vi "Hardware Out - NI 9759-1 (Throttle).vi"(0 "FPGA Ref":T3, 7 "ExternalAI1 (optional)":sgl, 9 "ExternalAI2 (optional)":sgl, 11 "RT Data in":T1={"Refs"={"FPGA 1"=refnum, "FPGA 2"=refnum}, "EPT"={"MaxCAD"=0.0, "EPT Sim Enabled"=FALSE, "EPTxData"={"Sync"=FALSE, "CurrentCAD"=0.0, "Speed [RPM]"=0.0, "Config"=FALSE, "Rcvg Primary"=FALSE, "Stall"=FALSE, "Overflow"=FALSE, "Ratio Error"=FALSE, "Pattern Error"=FALSE, "Aux Warning"=FALSE, "Watchdog Error"=FALSE}}, "Raw Inputs"={"NI9752s"=[], "NI9757s"=[], "NI9411s"=[], "NI9220s"=[], "VRHalls"=[]}, "Control Inputs"={"Engine Speed [RPM]"=0.0, "Engine Status"=enum."STALLED", "Load Control \nMode"=enum."Max Speed Governor", "dt(s)"=0.0, "Number of Cylinders"=0, "Engine Displacement [cc]"=0.0, "StoichAFR"=0.0, "Q.LHV Fuel [kJ/kg]"=0.0, "BattV PSU [V]"=0.0, "12V PSU [V]"=0.0, "5V PSU [V]"=0.0, "Pedal Position [%]"=0.0, "Oil Pressure [kPa]"=0.0, "Oil Temp [C]"=0.0, "Oil Level [%]"=0.0, "Engine Coolant Temp (ECT) [C]"=0.0, "Engine Coolant Pressure [kPa]"=0.0, "Rail Pressure [bar]"=0.0, "Fuel Pressure [kPa]"=0.0, "Fuel Temp [C]"=0.0, "Vacuum Pressure [kPa]"=0.0, "Throttle Position [%]"=0.0, "Cam1 Advance [CAD]"=0.0, "Cam2 Advance [CAD]"=0.0, "Cam3 Advance [CAD]"=0.0, "Cam4 Advance [CAD]"=0.0, "CA50 Control Output [CAD]"=[], "CA50 Control Output Valid"=[], "Intake Air Temp (IAT) [C]"=0.0, "Barometric Air Pressure [kPa]"=0.0, "Intake Air Rel. Humidity [%]"=0.0, "Mass Air Flow (MAF) [kg/hr]"=0.0, "Turbo Inlet Air Pressure [kPa]"=0.0, "Turbo Inlet Air Temp [C]"=0.0, "Turbo Outlet Air Pressure [kPa]"=0.0, "Turbo Outlet Air Temp [C]"=0.0, "CAC Outlet Pressure [kPa]"=0.0, "CAC Outlet Temp [C]"=0.0, "Intake Manifold Pressure (MAP) [kPa]"=0.0, "Intake Manifold Temp (MAT) [C]"=0.0, "Exhaust Manifold Pressure [kPa]"=0.0, "Exhaust Manifold Temp [C]"=0.0, "HighP EGR Cooler Outlet Pressure [kPa]"=0.0, "HighP EGR Cooler Outlet Temp [C]"=0.0, "HighP EGR Differential Pressure [kPa]"=0.0, "HighP EGR Valve Position [%]"=0.0, "Turbo Outlet Exhaust Pressure [kPa]"=0.0, "Turbo Outlet Exhaust Temp [C]"=0.0, "VGT Position 1 [%]"=0.0, "VGT Position 2 [%]"=0.0, "Turbo Speed 1 [RPM]"=0.0, "Turbo Speed 2 [RPM]"=0.0, "LowP EGR Differential Pressure [kPa]"=0.0, "LowP EGR Valve Position [%]"=0.0, "UEGO1Lambda"=0.0, "UEGO1_Hot"=FALSE, "UEGO2Lambda"=0.0, "UEGO2_Hot"=FALSE, "Knock Intensity"=[], "Knock"=[]}, "Control Outputs"={"Pedal Desired [%]"=0.0, "MEP Desired [bar]"=0.0, "Fuel Desired [mg/cyc]"=0.0, "Intake MAP Desired [kPa]"=0.0, "Cam1 Advance Setpoint [CAD]"=0.0, "Cam2 Advance Setpoint [CAD]"=0.0, "HighP EGR Position Setpoint [%Open]"=0.0, "LowP EGR Position Setpoint [%Open]"=0.0, "Rail Pressure Setpoint [bar]"=0.0, "Wastegate1 Position Setpoint [%Open]"=0.0, "Wastegate2 Position Setpoint [%Open]"=0.0, "VGT1 Position Setpoint [%Open]"=0.0, "VGT2 Position Setpoint [%Open]"=0.0, "Throttle1 Position Setpoint [%Open]"=0.0, "Throttle2 Position Setpoint [%Open]"=0.0, "TurboBPV Position Setpoint [%Open]"=0.0, "Spark Dwells [msec]"=[], "Spark Timings [DBTDC]"=[], "PFI Quantities [mg/inj]"=[], "PFI Timings [DBTDC]"=[], "DI Quantities [mg/inj]"=[], "DI Timings [DBTDC]"=[]}, "Raw Outputs"={"9751-1"={"DI1"={"Window_Start (DBTDC)"=0.0, "Window_End (DBTDC)"=0.0, "Enable_Inj1"=FALSE, "Duration_Inj1 (msec)"=0.0, "Timing_Inj1 (DBTDC)"=0.0, "Enable_Inj2"=FALSE, "Duration_Inj2 (msec)"=0.0, "Timing_Inj2 (DBTDC)"=0.0, "Enable_Inj3"=FALSE, "Duration_Inj3 (msec)"=0.0, "Timing_Inj3 (DBTDC)"=0.0, "Enable_Inj4"=FALSE, "Duration_Inj4 (msec)"=0.0, "Timing_Inj4 (DBTDC)"=0.0, "Enable_Inj5"=FALSE, "Duration_Inj5 (msec)"=0.0, "Timing_Inj5 (DBTDC)"=0.0}, "DI2"={"Window_Start (DBTDC)"=0.0, "Window_End (DBTDC)"=0.0, "Enable_Inj1"=FALSE, "Duration_Inj1 (msec)"=0.0, "Timing_Inj1 (DBTDC)"=0.0, "Enable_Inj2"=FALSE, "Duration_Inj2 (msec)"=0.0, "Timing_Inj2 (DBTDC)"=0.0, "Enable_Inj3"=FALSE, "Duration_Inj3 (msec)"=0.0, "Timing_Inj3 (DBTDC)"=0.0, "Enable_Inj4"=FALSE, "Duration_Inj4 (msec)"=0.0, "Timing_Inj4 (DBTDC)"=0.0, "Enable_Inj5"=FALSE, "Duration_Inj5 (msec)"=0.0, "Timing_Inj5 (DBTDC)"=0.0}, "DI3"={"Window_Start (DBTDC)"=0.0, "Window_End (DBTDC)"=0.0, "Enable_Inj1"=FALSE, "Duration_Inj1 (msec)"=0.0, "Timing_Inj1 (DBTDC)"=0.0, "Enable_Inj2"=FALSE, "Duration_Inj2 (msec)"=0.0, "Timing_Inj2 (DBTDC)"=0.0, "Enable_Inj3"=FALSE, "Duration_Inj3 (msec)"=0.0, "Timing_Inj3 (DBTDC)"=0.0, "Enable_Inj4"=FALSE, "Duration_Inj4 (msec)"=0.0, "Timing_Inj4 (DBTDC)"=0.0, "Enable_Inj5"=FALSE, "Duration_Inj5 (msec)"=0.0, "Timing_Inj5 (DBTDC)"=0.0}}, "9751-2"={"DI1"={"Window_Start (DBTDC)"=0.0, "Window_End (DBTDC)"=0.0, "Enable_Inj1"=FALSE, "Duration_Inj1 (msec)"=0.0, "Timing_Inj1 (DBTDC)"=0.0, "Enable_Inj2"=FALSE, "Duration_Inj2 (msec)"=0.0, "Timing_Inj2 (DBTDC)"=0.0, "Enable_Inj3"=FALSE, "Duration_Inj3 (msec)"=0.0, "Timing_Inj3 (DBTDC)"=0.0, "Enable_Inj4"=FALSE, "Duration_Inj4 (msec)"=0.0, "Timing_Inj4 (DBTDC)"=0.0, "Enable_Inj5"=FALSE, "Duration_Inj5 (msec)"=0.0, "Timing_Inj5 (DBTDC)"=0.0}, "DI2"={"Window_Start (DBTDC)"=0.0, "Window_End (DBTDC)"=0.0, "Enable_Inj1"=FALSE, "Duration_Inj1 (msec)"=0.0, "Timing_Inj1 (DBTDC)"=0.0, "Enable_Inj2"=FALSE, "Duration_Inj2 (msec)"=0.0, "Timing_Inj2 (DBTDC)"=0.0, "Enable_Inj3"=FALSE, "Duration_Inj3 (msec)"=0.0, "Timing_Inj3 (DBTDC)"=0.0, "Enable_Inj4"=FALSE, "Duration_Inj4 (msec)"=0.0, "Timing_Inj4 (DBTDC)"=0.0, "Enable_Inj5"=FALSE, "Duration_Inj5 (msec)"=0.0, "Timing_Inj5 (DBTDC)"=0.0}, "DI3"={"Window_Start (DBTDC)"=0.0, "Window_End (DBTDC)"=0.0, "Enable_Inj1"=FALSE, "Duration_Inj1 (msec)"=0.0, "Timing_Inj1 (DBTDC)"=0.0, "Enable_Inj2"=FALSE, "Duration_Inj2 (msec)"=0.0, "Timing_Inj2 (DBTDC)"=0.0, "Enable_Inj3"=FALSE, "Duration_Inj3 (msec)"=0.0, "Timing_Inj3 (DBTDC)"=0.0, "Enable_Inj4"=FALSE, "Duration_Inj4 (msec)"=0.0, "Timing_Inj4 (DBTDC)"=0.0, "Enable_Inj5"=FALSE, "Duration_Inj5 (msec)"=0.0, "Timing_Inj5 (DBTDC)"=0.0}}, "9751-3"={"DI1"={"Window_Start (DBTDC)"=0.0, "Window_End (DBTDC)"=0.0, "Enable_Inj1"=FALSE, "Duration_Inj1 (msec)"=0.0, "Timing_Inj1 (DBTDC)"=0.0, "Enable_Inj2"=FALSE, "Duration_Inj2 (msec)"=0.0, "Timing_Inj2 (DBTDC)"=0.0, "Enable_Inj3"=FALSE, "Duration_Inj3 (msec)"=0.0, "Timing_Inj3 (DBTDC)"=0.0, "Enable_Inj4"=FALSE, "Duration_Inj4 (msec)"=0.0, "Timing_Inj4 (DBTDC)"=0.0, "Enable_Inj5"=FALSE, "Duration_Inj5 (msec)"=0.0, "Timing_Inj5 (DBTDC)"=0.0}, "DI2"={"Window_Start (DBTDC)"=0.0, "Window_End (DBTDC)"=0.0, "Enable_Inj1"=FALSE, "Duration_Inj1 (msec)"=0.0, "Timing_Inj1 (DBTDC)"=0.0, "Enable_Inj2"=FALSE, "Duration_Inj2 (msec)"=0.0, "Timing_Inj2 (DBTDC)"=0.0, "Enable_Inj3"=FALSE, "Duration_Inj3 (msec)"=0.0, "Timing_Inj3 (DBTDC)"=0.0, "Enable_Inj4"=FALSE, "Duration_Inj4 (msec)"=0.0, "Timing_Inj4 (DBTDC)"=0.0, "Enable_Inj5"=FALSE, "Duration_Inj5 (msec)"=0.0, "Timing_Inj5 (DBTDC)"=0.0}, "DI3"={"Window_Start (DBTDC)"=0.0, "Window_End (DBTDC)"=0.0, "Enable_Inj1"=FALSE, "Duration_Inj1 (msec)"=0.0, "Timing_Inj1 (DBTDC)"=0.0, "Enable_Inj2"=FALSE, "Duration_Inj2 (msec)"=0.0, "Timing_Inj2 (DBTDC)"=0.0, "Enable_Inj3"=FALSE, "Duration_Inj3 (msec)"=0.0, "Timing_Inj3 (DBTDC)"=0.0, "Enable_Inj4"=FALSE, "Duration_Inj4 (msec)"=0.0, "Timing_Inj4 (DBTDC)"=0.0, "Enable_Inj5"=FALSE, "Duration_Inj5 (msec)"=0.0, "Timing_Inj5 (DBTDC)"=0.0}}, "9751-4"={"DI1"={"Window_Start (DBTDC)"=0.0, "Window_End (DBTDC)"=0.0, "Enable_Inj1"=FALSE, "Duration_Inj1 (msec)"=0.0, "Timing_Inj1 (DBTDC)"=0.0, "Enable_Inj2"=FALSE, "Duration_Inj2 (msec)"=0.0, "Timing_Inj2 (DBTDC)"=0.0, "Enable_Inj3"=FALSE, "Duration_Inj3 (msec)"=0.0, "Timing_Inj3 (DBTDC)"=0.0, "Enable_Inj4"=FALSE, "Duration_Inj4 (msec)"=0.0, "Timing_Inj4 (DBTDC)"=0.0, "Enable_Inj5"=FALSE, "Duration_Inj5 (msec)"=0.0, "Timing_Inj5 (DBTDC)"=0.0}, "DI2"={"Window_Start (DBTDC)"=0.0, "Window_End (DBTDC)"=0.0, "Enable_Inj1"=FALSE, "Duration_Inj1 (msec)"=0.0, "Timing_Inj1 (DBTDC)"=0.0, "Enable_Inj2"=FALSE, "Duration_Inj2 (msec)"=0.0, "Timing_Inj2 (DBTDC)"=0.0, "Enable_Inj3"=FALSE, "Duration_Inj3 (msec)"=0.0, "Timing_Inj3 (DBTDC)"=0.0, "Enable_Inj4"=FALSE, "Duration_Inj4 (msec)"=0.0, "Timing_Inj4 (DBTDC)"=0.0, "Enable_Inj5"=FALSE, "Duration_Inj5 (msec)"=0.0, "Timing_Inj5 (DBTDC)"=0.0}, "DI3"={"Window_Start (DBTDC)"=0.0, "Window_End (DBTDC)"=0.0, "Enable_Inj1"=FALSE, "Duration_Inj1 (msec)"=0.0, "Timing_Inj1 (DBTDC)"=0.0, "Enable_Inj2"=FALSE, "Duration_Inj2 (msec)"=0.0, "Timing_Inj2 (DBTDC)"=0.0, "Enable_Inj3"=FALSE, "Duration_Inj3 (msec)"=0.0, "Timing_Inj3 (DBTDC)"=0.0, "Enable_Inj4"=FALSE, "Duration_Inj4 (msec)"=0.0, "Timing_Inj4 (DBTDC)"=0.0, "Enable_Inj5"=FALSE, "Duration_Inj5 (msec)"=0.0, "Timing_Inj5 (DBTDC)"=0.0}}, "9754-1"={"ESTTL 1"={"Timing (DBTDC)"=0.0, "Dwell (ms)"=0.0}, "ESTTL 2"={"Timing (DBTDC)"=0.0, "Dwell (ms)"=0.0}, "ESTTL 3"={"Timing (DBTDC)"=0.0, "Dwell (ms)"=0.0}, "ESTTL 4"={"Timing (DBTDC)"=0.0, "Dwell (ms)"=0.0}, "ESTTL 5"={"Timing (DBTDC)"=0.0, "Dwell (ms)"=0.0}, "ESTTL 6"={"Timing (DBTDC)"=0.0, "Dwell (ms)"=0.0}, "ESTTL 7"={"Timing (DBTDC)"=0.0, "Dwell (ms)"=0.0}, "ESTTL 8"={"Timing (DBTDC)"=0.0, "Dwell (ms)"=0.0}}, "9754-2"={"ESTTL 1"={"Timing (DBTDC)"=0.0, "Dwell (ms)"=0.0}, "ESTTL 2"={"Timing (DBTDC)"=0.0, "Dwell (ms)"=0.0}, "ESTTL 3"={"Timing (DBTDC)"=0.0, "Dwell (ms)"=0.0}, "ESTTL 4"={"Timing (DBTDC)"=0.0, "Dwell (ms)"=0.0}, "ESTTL 5"={"Timing (DBTDC)"=0.0, "Dwell (ms)"=0.0}, "ESTTL 6"={"Timing (DBTDC)"=0.0, "Dwell (ms)"=0.0}, "ESTTL 7"={"Timing (DBTDC)"=0.0, "Dwell (ms)"=0.0}, "ESTTL 8"={"Timing (DBTDC)"=0.0, "Dwell (ms)"=0.0}}, "9758-1"={"LS 1"={"Enable"=FALSE, "Freq [Hz]"=0.0, "DutyCyc [%]"=0.0}, "LS 2"={"Enable"=FALSE, "Freq [Hz]"=0.0, "DutyCyc [%]"=0.0}, "LS 3"={"Enable"=FALSE, "Freq [Hz]"=0.0, "DutyCyc [%]"=0.0}, "LS 4"={"Enable"=FALSE, "Freq [Hz]"=0.0, "DutyCyc [%]"=0.0}, "PFI 1"={"Position Mode"=FALSE, "Timing (DBTDC)"=0.0, "Pulse Width (ms)"=0.0}, "PFI 2"={"Position Mode"=FALSE, "Timing (DBTDC)"=0.0, "Pulse Width (ms)"=0.0}, "PFI 3"={"Position Mode"=FALSE, "Timing (DBTDC)"=0.0, "Pulse Width (ms)"=0.0}, "PFI 4"={"Position Mode"=FALSE, "Timing (DBTDC)"=0.0, "Pulse Width (ms)"=0.0}}, "9758-2"={"LS 1"={"Enable"=FALSE, "Freq [Hz]"=0.0, "DutyCyc [%]"=0.0}, "LS 2"={"Enable"=FALSE, "Freq [Hz]"=0.0, "DutyCyc [%]"=0.0}, "LS 3"={"Enable"=FALSE, "Freq [Hz]"=0.0, "DutyCyc [%]"=0.0}, "LS 4"={"Enable"=FALSE, "Freq [Hz]"=0.0, "DutyCyc [%]"=0.0}, "PFI 1"={"Position Mode"=FALSE, "Timing (DBTDC)"=0.0, "Pulse Width (ms)"=0.0}, "PFI 2"={"Position Mode"=FALSE, "Timing (DBTDC)"=0.0, "Pulse Width (ms)"=0.0}, "PFI 3"={"Position Mode"=FALSE, "Timing (DBTDC)"=0.0, "Pulse Width (ms)"=0.0}, "PFI 4"={"Position Mode"=FALSE, "Timing (DBTDC)"=0.0, "Pulse Width (ms)"=0.0}}, "9759-1"={"THR1-1 DC [%]"=0.0, "THR1-1 Setpoint [% Open]"=0.0, "THR1-2 DC [%]"=0.0, "THR1-2 Setpoint [% Open]"=0.0}}} {"Control Inputs"."Knock Intensity" format="%.2f"; "Control Inputs"."CA50 Control Output [CAD]" format="%.2f"; "Control Inputs"."Exhaust Manifold Temp [C]" format="%#_6f"; "Control Inputs"."UEGO2Lambda" format="%.2f"; "Control Inputs"."Intake Manifold Temp (MAT) [C]" format="%#_6f"; "Control Inputs"."UEGO1Lambda" format="%.2f"}) -> ()   [LabVIEW 2015, in "ECS-RT.lvlib"]
uses:
  ECS-RT.lvlib
  Typedefs/FPGA Refs/Generic FPGA Ref.ctl
  Typedefs/RT Data.ctl
  Typedefs/FPGA Refs/FPGA Refs.ctl
  Typedefs/EPT/EPT Cluster.ctl
  <vilib>/Powertrain Controls/Device Drivers/Engine Position Tracking/EPTx/RevA/RT/Controls/EPTxData.ctl
  Typedefs/Raw Inputs/Raw Inputs.ctl
  Typedefs/Raw Inputs/NI9752.ctl
  Typedefs/Raw Inputs/PPWData.ctl
  Typedefs/Raw Inputs/NI9757.ctl
  Typedefs/Raw Inputs/NI9411.ctl
  Typedefs/Raw Inputs/NI9220.ctl
  Typedefs/Raw Inputs/VRHall.ctl
  Typedefs/Control Inputs/Control Inputs.ctl
  Typedefs/EPT/Engine Status.ctl
  Typedefs/MISC/Load Control Mode.ctl
  Typedefs/Control Outputs/Control Outputs.ctl
  Typedefs/Control Outputs/Injection Quantity.ctl
  Typedefs/Control Outputs/Injection Timing.ctl
  Typedefs/Raw Outputs/Raw Outputs.ctl
  Typedefs/Raw Outputs/NI9751.ctl
  Typedefs/Raw Outputs/DI.ctl
  Typedefs/Raw Outputs/NI9754.ctl
  Typedefs/Raw Outputs/ESTTL.ctl
  Typedefs/Raw Outputs/NI9758.ctl
  Typedefs/Raw Outputs/LS.ctl
  Typedefs/Raw Outputs/PFI.ctl
  Typedefs/Raw Outputs/NI9759.ctl
  <vilib>/Powertrain Controls/Device Drivers/Throttle/RevB2/Real-Time/Support/Mode Request.ctl
  <vilib>/Utility/error.llb/Error Cluster From Error Code.vi
  <vilib>/rvi/errors/niLvFpgaAdjustHostInterfaceError.vi
  <vilib>/rvi/interface/nirviReadWriteControl/nirviReadWriteControl.xnode
  <vilib>/rvi/interface/Simulation/niFpgaSimulationCallBeginRW.vi
  NiFpgaLv.dll
  ECS-Shared.lvlib
  <vilib>/Powertrain Controls/Device Drivers/Engine Position Tracking/EPTx/RevA/RT/EPTx - RevA - RT.lvlib
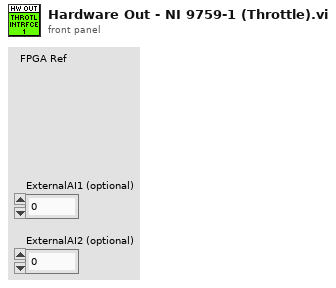
[diagram p1: front panel]
types:
  T1 = typedef "ECS-Shared.lvlib/RT Data.ctl" = cluster{"Refs":T2, "EPT":T4, "Raw Inputs":T6, "Control Inputs":T13, "Control Outputs":T16, "Raw Outputs":T19}
  T2 = typedef "ECS-Shared.lvlib/FPGA Refs.ctl" = cluster{"FPGA 1":T3, "FPGA 2":T3}
  T3 = typedef "ECS-Shared.lvlib/Generic FPGA Ref.ctl" = refnum<k20>
  T4 = typedef "ECS-Shared.lvlib/EPT Cluster.ctl" = cluster{"MaxCAD":sgl, "EPT Sim Enabled":bool, "EPTxData":T5}
  T5 = typedef "EPTx - RevA - RT.lvlib/EPTxData.ctl" = cluster{"Sync":bool, "CurrentCAD":sgl, "Speed [RPM]":sgl, "Config":bool, "Rcvg Primary":bool, "Stall":bool, "Overflow":bool, "Ratio Error":bool, "Pattern Error":bool, "Aux Warning":bool, "Watchdog Error":bool}
  T6 = typedef "ECS-Shared.lvlib/Raw Inputs.ctl" = cluster{"NI9752s":T7[], "NI9757s":T9[], "NI9411s":T10[], "NI9220s":T11[], "VRHalls":T12[]}
  T7 = typedef "ECS-Shared.lvlib/NI9752.ctl" = cluster{"Voltage [V]":sgl[], "Resistance [Ohm]":sgl[], "PPWData VR1":T8, "PPWData VR2":T8, "PPWData Hall1":T8, "PPWData Hall2":T8}
  T8 = typedef "ECS-Shared.lvlib/PPWData.ctl" = cluster{"Period":u32, "PulseWidth":u32, "Stopped":bool}
  T9 = typedef "ECS-Shared.lvlib/NI9757.ctl" = cluster{"UEGO1":cluster{"Lambda":sgl, "Phi":sgl, "AF_Ratio":sgl, "Ip":sgl, "Temp":sgl, "Hot":bool}, "UEGO2":cluster{"Lambda":sgl, "Phi":sgl, "AF_Ratio":sgl, "Ip":sgl, "Temp":sgl, "Hot":bool}, "EGO1":cluster{"Status":enum16{"COLD SENSOR", "FOULED SENSOR", "RICH", "LEAN"}, "SensorV":sgl}, "EGO2":cluster{"Status":enum16{"COLD SENSOR", "FOULED SENSOR", "RICH", "LEAN"}, "SensorV":sgl}, "EGO3":cluster{"Status":enum16{"COLD SENSOR", "FOULED SENSOR", "RICH", "LEAN"}, "SensorV":sgl}, "EGO4":cluster{"Status":enum16{"COLD SENSOR", "FOULED SENSOR", "RICH", "LEAN"}, "SensorV":sgl}}
  T10 = typedef "ECS-Shared.lvlib/NI9411.ctl" = cluster{"PPWData 0":T8, "PPWData 1":T8, "PPWData 2":T8, "PPWData 3":T8, "PPWData 4":T8, "PPWData 5":T8}
  T11 = typedef "ECS-Shared.lvlib/NI9220.ctl" = cluster{"AI 0":sgl, "AI 1":sgl, "AI 2":sgl, "AI 3":sgl, "AI 4":sgl, "AI 5":sgl, "AI 6":sgl, "AI 7":sgl, "AI 8":sgl, "AI 9":sgl, "AI 10":sgl, "AI 11":sgl, "AI 12":sgl, "AI 13":sgl, "AI 14":sgl, "AI 15":sgl}
  T12 = typedef "ECS-Shared.lvlib/VRHall.ctl" = cluster{"PPWData 0":T8, "PPWData 1":T8, "PPWData 2":T8, "PPWData 3":T8, "PPWData 4":T8, "PPWData 5":T8}
  T13 = typedef "ECS-Shared.lvlib/Control Inputs.ctl" = cluster{"Engine Speed [RPM]":sgl, "Engine Status":T14, "Load Control \nMode":T15, "dt(s)":sgl, "Number of Cylinders":u8, "Engine Displacement [cc]":sgl, "StoichAFR":sgl, "Q.LHV Fuel [kJ/kg]":sgl, "BattV PSU [V]":sgl, "12V PSU [V]":sgl, "5V PSU [V]":sgl, "Pedal Position [%]":sgl, "Oil Pressure [kPa]":sgl, "Oil Temp [C]":sgl, "Oil Level [%]":sgl, "Engine Coolant Temp (ECT) [C]":sgl, "Engine Coolant Pressure [kPa]":sgl, "Rail Pressure [bar]":sgl, "Fuel Pressure [kPa]":sgl, "Fuel Temp [C]":sgl, "Vacuum Pressure [kPa]":sgl, "Throttle Position [%]":sgl, "Cam1 Advance [CAD]":sgl, "Cam2 Advance [CAD]":sgl, "Cam3 Advance [CAD]":sgl, "Cam4 Advance [CAD]":sgl, "CA50 Control Output [CAD]":sgl[], "CA50 Control Output Valid":bool[], "Intake Air Temp (IAT) [C]":sgl, "Barometric Air Pressure [kPa]":sgl, "Intake Air Rel. Humidity [%]":sgl, "Mass Air Flow (MAF) [kg/hr]":sgl, "Turbo Inlet Air Pressure [kPa]":sgl, "Turbo Inlet Air Temp [C]":sgl, "Turbo Outlet Air Pressure [kPa]":sgl, "Turbo Outlet Air Temp [C]":sgl, "CAC Outlet Pressure [kPa]":sgl, "CAC Outlet Temp [C]":sgl, "Intake Manifold Pressure (MAP) [kPa]":sgl, "Intake Manifold Temp (MAT) [C]":sgl, "Exhaust Manifold Pressure [kPa]":sgl, "Exhaust Manifold Temp [C]":sgl, "HighP EGR Cooler Outlet Pressure [kPa]":sgl, "HighP EGR Cooler Outlet Temp [C]":sgl, "HighP EGR Differential Pressure [kPa]":sgl, "HighP EGR Valve Position [%]":sgl, "Turbo Outlet Exhaust Pressure [kPa]":sgl, "Turbo Outlet Exhaust Temp [C]":sgl, "VGT Position 1 [%]":sgl, "VGT Position 2 [%]":sgl, "Turbo Speed 1 [RPM]":sgl, "Turbo Speed 2 [RPM]":sgl, "LowP EGR Differential Pressure [kPa]":sgl, "LowP EGR Valve Position [%]":sgl, "UEGO1Lambda":sgl, "UEGO1_Hot":bool, "UEGO2Lambda":sgl, "UEGO2_Hot":bool, "Knock Intensity":sgl[], "Knock":bool[]}
  T14 = typedef "ECS-Shared.lvlib/Engine Status.ctl" = enum16{"OFF", "STALLED", "CRANKING", "RUNNING", "ACCEL", "DECEL", "SAFE"}
  T15 = typedef "ECS-Shared.lvlib/Load Control Mode.ctl" = enum16{"No Governor", "Min Speed Governor", "Max Speed Governor"}
  T16 = typedef "ECS-Shared.lvlib/Control Outputs.ctl" = cluster{"Pedal Desired [%]":sgl, "MEP Desired [bar]":sgl, "Fuel Desired [mg/cyc]":sgl, "Intake MAP Desired [kPa]":sgl, "Cam1 Advance Setpoint [CAD]":sgl, "Cam2 Advance Setpoint [CAD]":sgl, "HighP EGR Position Setpoint [%Open]":sgl, "LowP EGR Position Setpoint [%Open]":sgl, "Rail Pressure Setpoint [bar]":sgl, "Wastegate1 Position Setpoint [%Open]":sgl, "Wastegate2 Position Setpoint [%Open]":sgl, "VGT1 Position Setpoint [%Open]":sgl, "VGT2 Position Setpoint [%Open]":sgl, "Throttle1 Position Setpoint [%Open]":sgl, "Throttle2 Position Setpoint [%Open]":sgl, "TurboBPV Position Setpoint [%Open]":sgl, "Spark Dwells [msec]":sgl[], "Spark Timings [DBTDC]":sgl[], "PFI Quantities [mg/inj]":sgl[], "PFI Timings [DBTDC]":sgl[], "DI Quantities [mg/inj]":T17[], "DI Timings [DBTDC]":T18[]}
  T17 = typedef "ECS-Shared.lvlib/Injection Quantity.ctl" = cluster{"Pilot1Quantity [mg/inj]":sgl, "Pilot2Quantity [mg/inj]":sgl, "MainQuantity [mg/inj]":sgl, "Post1Quantity [mg/inj]":sgl, "Post2Quantity [mg/inj]":sgl}
  T18 = typedef "ECS-Shared.lvlib/Injection Timing.ctl" = cluster{"Pilot1SOI [DBTDC]":sgl, "Pilot2SOI [DBTDC]":sgl, "MainSOI [DBTDC]":sgl, "Post1SOI [DBTDC]":sgl, "Post2SOI [DBTDC]":sgl}
  T19 = typedef "ECS-Shared.lvlib/Raw Outputs.ctl" = cluster{"9751-1":T20, "9751-2":T20, "9751-3":T20, "9751-4":T20, "9754-1":T22, "9754-2":T22, "9758-1":T24, "9758-2":T24, "9759-1":T27}
  T20 = typedef "ECS-Shared.lvlib/NI9751.ctl" = cluster{"DI1":T21, "DI2":T21, "DI3":T21}
  T21 = typedef "ECS-Shared.lvlib/DI.ctl" = cluster{"Window_Start (DBTDC)":sgl, "Window_End (DBTDC)":sgl, "Enable_Inj1":bool, "Duration_Inj1 (msec)":sgl, "Timing_Inj1 (DBTDC)":sgl, "Enable_Inj2":bool, "Duration_Inj2 (msec)":sgl, "Timing_Inj2 (DBTDC)":sgl, "Enable_Inj3":bool, "Duration_Inj3 (msec)":sgl, "Timing_Inj3 (DBTDC)":sgl, "Enable_Inj4":bool, "Duration_Inj4 (msec)":sgl, "Timing_Inj4 (DBTDC)":sgl, "Enable_Inj5":bool, "Duration_Inj5 (msec)":sgl, "Timing_Inj5 (DBTDC)":sgl}
  T22 = typedef "ECS-Shared.lvlib/NI9754.ctl" = cluster{"ESTTL 1":T23, "ESTTL 2":T23, "ESTTL 3":T23, "ESTTL 4":T23, "ESTTL 5":T23, "ESTTL 6":T23, "ESTTL 7":T23, "ESTTL 8":T23}
  T23 = typedef "ECS-Shared.lvlib/ESTTL.ctl" = cluster{"Timing (DBTDC)":sgl, "Dwell (ms)":sgl}
  T24 = typedef "ECS-Shared.lvlib/NI9758.ctl" = cluster{"LS 1":T25, "LS 2":T25, "LS 3":T25, "LS 4":T25, "PFI 1":T26, "PFI 2":T26, "PFI 3":T26, "PFI 4":T26}
  T25 = typedef "ECS-Shared.lvlib/LS.ctl" = cluster{"Enable":bool, "Freq [Hz]":sgl, "DutyCyc [%]":sgl}
  T26 = typedef "ECS-Shared.lvlib/PFI.ctl" = cluster{"Position Mode":bool, "Timing (DBTDC)":sgl, "Pulse Width (ms)":sgl}
  T27 = typedef "ECS-Shared.lvlib/NI9759.ctl" = cluster{"THR1-1 DC [%]":sgl, "THR1-1 Setpoint [% Open]":sgl, "THR1-2 DC [%]":sgl, "THR1-2 Setpoint [% Open]":sgl}
  T28 = cluster{"TLead (sec)":sgl, "TLag (sec)":sgl, "KRpos (V/ )":sgl, "TIpos (sec)":sgl, "TDpos (sec)":sgl, "KRneg (V/ )":sgl, "TIneg (sec)":sgl, "TDneg (sec)":sgl, "LH Position Band":sgl, "U LH (V)":sgl, "U LH Lag (sec)":sgl, "US (V)":sgl, "US Lag (sec)":sgl, "LH Position":sgl, "Motor Resistance (Ohms)":sgl, "Position Fault Thresh":sgl}
  T29 = typedef "Mode Request.ctl" = enum16{"IDLE", "POSITION CALIBRATION", "CONTROL CALIBRATION", "CONTROL"}
  T30 = cluster{"Analog1 Range (V)":sgl[], "Analog2 Range (V)":sgl[], "Position Range":sgl[]}
  T31 = cluster{"Psn Cal Init Delay (sec)":sgl, "Psn Cal Return From Postive Delay (sec)":sgl, "Psn Cal Return From Negative Delay (sec)":sgl, "u Psn Cal Postive Init (V)":sgl, "u Psn Cal Negative Init (V)":sgl, "u Psn Cal Inc (V)":sgl, "u Psn Cal Dec (V)":sgl, "u Psn Cal Inc Thresh (V)":sgl, "u Psn Cal Dec Thresh (V)":sgl, "Psn Cal Offset (V)":sgl, "Psn Cal Diff Thresh (V)":sgl}
  T32 = cluster{"ModuleEnable":bool, "WatchdogIn":bool, "ThrottlePeriod":u16, "Throttle2Period":u16, "ThrottlePulseWidth":i16, "Throttle2PulseWidth":i16}
  T33 = cluster{"ModulePresent":bool, "H1Sense":i16, "H2Sense":i16, "Analog1":i16, "Analog2":i16, "Battery":i16, "Temperature":i16, "Fault1":bool, "Fault2":bool}
  T34 = cluster{"ModulePresent":bool, "H1Sense (A)":sgl, "H2Sense (A)":sgl, "Analog1 (V)":sgl, "Analog2 (V)":sgl, "Battery (V)":sgl, "Temperature (C)":sgl, "H1Fault":bool, "H2Fault":bool}
  T35 = cluster{"Primary Analog Range (V)":sgl[], "Secondary Analog Range (V)":sgl[], "Position Range":sgl[], "Position Calibrated":bool, "u Pos Cal Positive (V)":sgl, "u Pos Cal Negative (V)":sgl, "u Limit Positive":bool, "u Limit Negative":bool, "Pos Cal Diff Fault":bool}
  T36 = typedef "Mode Status.ctl" = enum16{"IDLE", "POSITION CALIBRATION", "CONTROL CALIBRATION", "CONTROL"}
  T37 = cluster{"Primary Position":sgl, "Secondary Position":sgl, "AboveLH?":bool, "Position Fault":bool, "u Limit?":bool, "uLHc (V)":sgl, "uFc (V)":sgl, "uPID (V)":sgl, "u (V)":sgl}
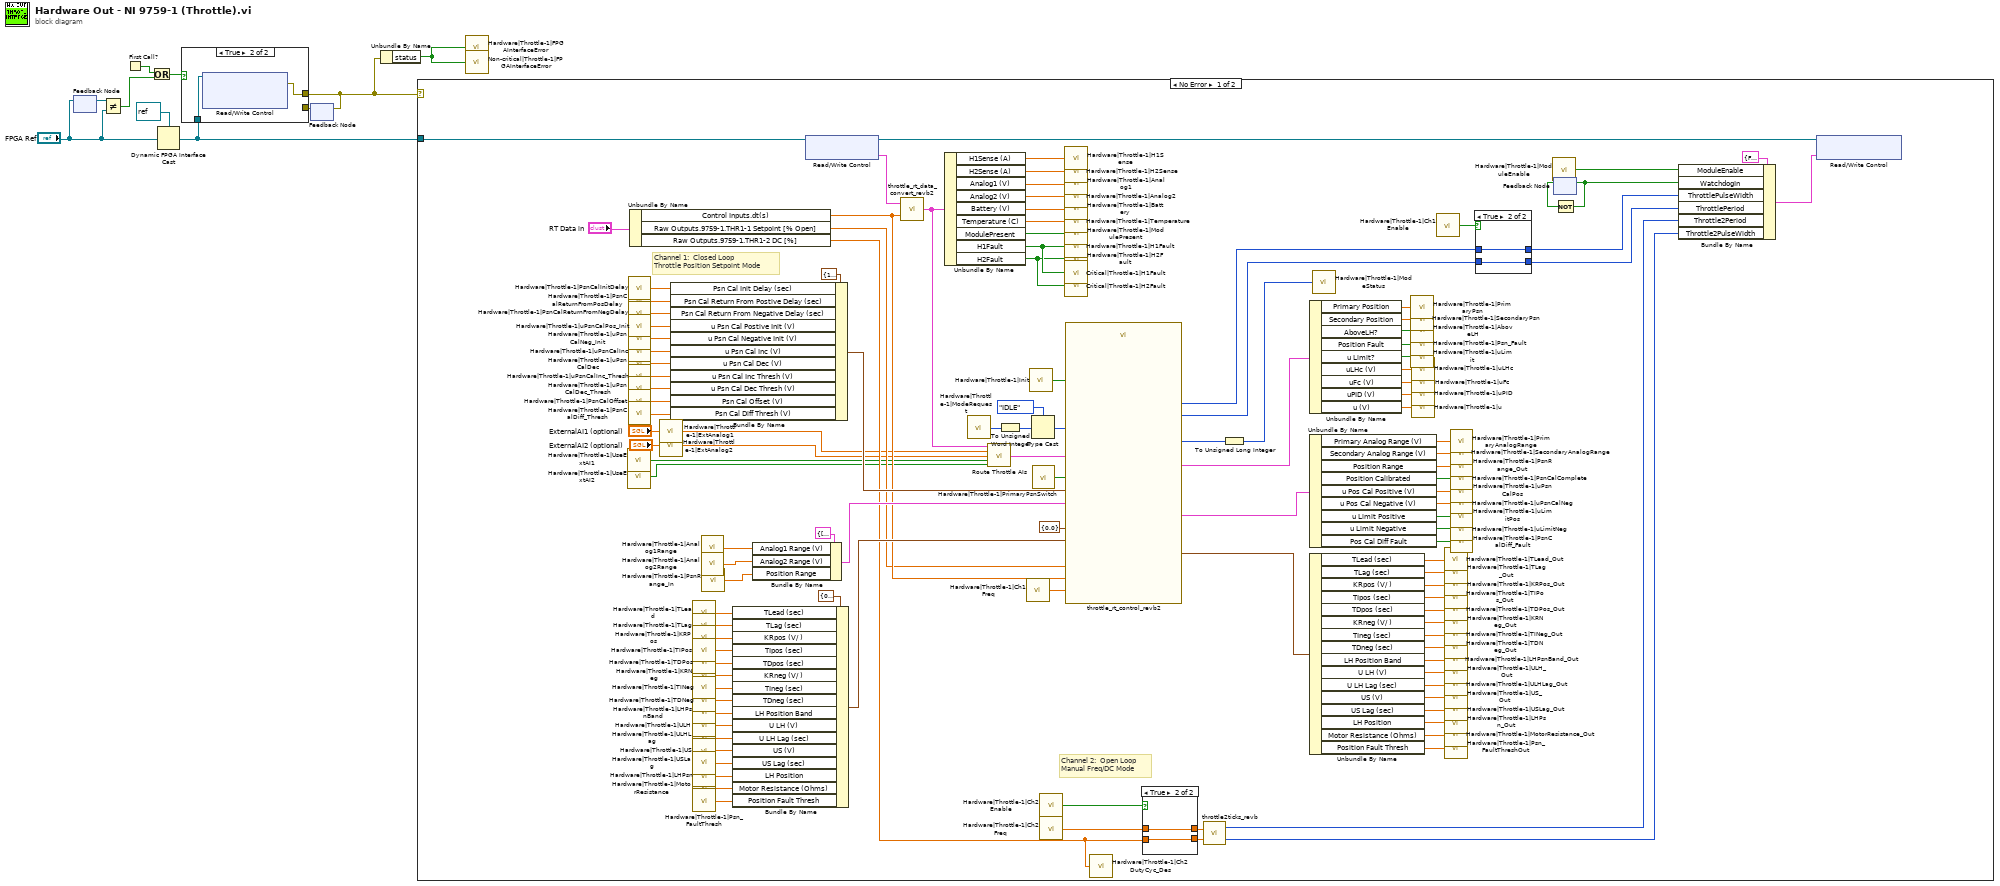
[diagram p0: block diagram]
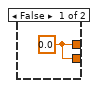
[diagram p3: hidden frame]
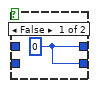
[diagram p4: hidden frame]
diagram:
  n1 = feedback #1() -> (w7:T3)  [unwired: 1 in]
  n2 = feedback-in #1("FPGA Ref") -> ()
  n3 = Not Equal?(x=w7, y="FPGA Ref") -> (x != y?=w6:bool)
  n4 = First Call?() -> (First Call?: T/F=w8:bool)
  n5 = Or(x=w8, y=w6) -> (x .or. y?=w9:bool)
  n6 = Dynamic FPGA Interface Cast(Session In=refnum<k20> refnum ("NI 9759 (Throttle)"), Type="FPGA Ref") -> (Session Out=w5:refnum<k20>)
  n7 = feedback #2() -> (w10:errorcluster)  [unwired: 1 in]
  n8 = case shown="True" w9 {
    tunnel: [w11 w13] -> w2
    tunnel: w10 -> [w11 _]
    tunnel: w5 -> [_ w12]
    frame False {
    }
    frame True {
      n9 = xnode "Read/Write Control"("FPGA VI Reference In"=w12) -> ("error out"=w13:errorcluster)  [unwired: 2 in, 2 out]
    }
  }
  n10 = feedback-in #2(w2) -> ()
  n11 = Unbundle By Name(w2) -> ("status"=w1:bool)
  n12 = case shown="No Error" w2 {
    tunnel: w5 -> [w27 _]
    frame No Error {
      # "Channel 2:  Open Loop\nManual Freq/DC Mode"
      # "Channel 1:  Closed Loop\nThrottle Position Setpoint Mode"
      n13 = call "Hardware|Throttle-1|UseExtAI1"() -> ("Value"=w17:bool)
      n14 = call "Hardware|Throttle-1|UseExtAI2"() -> ("Value"=w16:bool)
      n15 = call "Hardware|Throttle-1|PsnCalInitDelay"() -> ("Value"=w106:sgl)
      n16 = call "Hardware|Throttle-1|PsnCalReturnFromPosDelay"() -> ("Value"=w104:sgl)
      n17 = call "Hardware|Throttle-1|PsnCalReturnFromNegDelay"() -> ("Value"=w103:sgl)
      n18 = call "Hardware|Throttle-1|uPsnCalPos_Init"() -> ("Value"=w102:sgl)
      n19 = call "Hardware|Throttle-1|uPsnCalNeg_Init"() -> ("Value"=w101:sgl)
      n20 = call "Hardware|Throttle-1|uPsnCalInc"() -> ("Value"=w100:sgl)
      n21 = call "Hardware|Throttle-1|uPsnCalDec"() -> ("Value"=w99:sgl)
      n22 = call "Hardware|Throttle-1|uPsnCalInc_Thresh"() -> ("Value"=w98:sgl)
      n23 = call "Hardware|Throttle-1|uPsnCalDec_Thresh"() -> ("Value"=w97:sgl)
      n24 = call "Hardware|Throttle-1|PsnCalOffset"() -> ("Value"=w96:sgl)
      n25 = call "Hardware|Throttle-1|PsnCalDiff_Thresh"() -> ("Value"=w105:sgl)
      n26 = Unbundle By Name("RT Data in") -> ("Control Inputs.dt(s)"=w23:sgl, "Raw Outputs.9759-1.THR1-1 Setpoint [% Open]"=w22:sgl, "Raw Outputs.9759-1.THR1-2 DC [%]"=w21:sgl)
      n27 = call "Hardware|Throttle-1|ExtAnalog1"("Value"="ExternalAI1 (optional)") -> ()
      n28 = call "Hardware|Throttle-1|ExtAnalog2"("Value"="ExternalAI2 (optional)") -> ()
      n29 = Bundle By Name(cluster=T31 {"Psn Cal Init Delay (sec)"=1.0, "Psn Cal Return From Postive Delay (sec)"=1.0, "Psn Cal Return From Negative Delay (sec)"=1.0, "u Psn Cal Postive Init (V)"=3.4, "u Psn Cal Negative Init (V)"=-3.0, "u Psn Cal Inc (V)"=0.2, "u Psn Cal Dec (V)"=-0.2, "u Psn Cal Inc Thresh (V)"=1.1, "u Psn Cal Dec Thresh (V)"=-1.1, "Psn Cal Offset (V)"=0.005, "Psn Cal Diff Thresh (V)"=3.0} ("Position Cal Settings"), "Psn Cal Init Delay (sec)"=w106, "Psn Cal Return From Postive Delay (sec)"=w104, "Psn Cal Return From Negative Delay (sec)"=w103, "u Psn Cal Postive Init (V)"=w102, "u Psn Cal Negative Init (V)"=w101, "u Psn Cal Inc (V)"=w100, "u Psn Cal Dec (V)"=w99, "u Psn Cal Inc Thresh (V)"=w98, "u Psn Cal Dec Thresh (V)"=w97, "Psn Cal Offset (V)"=w96, "Psn Cal Diff Thresh (V)"=w105) -> (w112:T31)
      n30 = call "Hardware|Throttle-1|TLead"() -> ("Value"=w114:sgl)
      n31 = call "Hardware|Throttle-1|TLag"() -> ("Value"=w115:sgl)
      n32 = call "Hardware|Throttle-1|KRPos"() -> ("Value"=w116:sgl)
      n33 = call "Hardware|Throttle-1|TIPos"() -> ("Value"=w117:sgl)
      n34 = call "Hardware|Throttle-1|TDPos"() -> ("Value"=w118:sgl)
      n35 = call "Hardware|Throttle-1|KRNeg"() -> ("Value"=w119:sgl)
      n36 = call "Hardware|Throttle-1|TINeg"() -> ("Value"=w120:sgl)
      n37 = call "Hardware|Throttle-1|TDNeg"() -> ("Value"=w121:sgl)
      n38 = call "Hardware|Throttle-1|LHPsnBand"() -> ("Value"=w122:sgl)
      n39 = call "Hardware|Throttle-1|ULH"() -> ("Value"=w123:sgl)
      n40 = call "Hardware|Throttle-1|ULHLag"() -> ("Value"=w124:sgl)
      n41 = call "Hardware|Throttle-1|US"() -> ("Value"=w52:sgl)
      n42 = call "Hardware|Throttle-1|USLag"() -> ("Value"=w51:sgl)
      n43 = call "Hardware|Throttle-1|LHPsn"() -> ("Value"=w50:sgl)
      n44 = call "Hardware|Throttle-1|MotorResistance"() -> ("Value"=w49:sgl)
      n45 = call "Hardware|Throttle-1|Psn_FaultThresh"() -> ("Value"=w29:sgl)
      n46 = call "Hardware|Throttle-1|Analog1Range"() -> ("Value"=w95:sgl[])
      n47 = call "Hardware|Throttle-1|Analog2Range"() -> ("Value"=w94:sgl[])
      n48 = call "Hardware|Throttle-1|PsnRange_In"() -> ("Value"=w93:sgl[])
      n49 = Bundle By Name(cluster=T28 {"TLead (sec)"=0.0, "TLag (sec)"=0.1, "KRpos (V/ )"=0.5, "TIpos (sec)"=0.15, "TDpos (sec)"=0.01, "KRneg (V/ )"=1.0, "TIneg (sec)"=0.1, "TDneg (sec)"=0.001, "LH Position Band"=0.2, "U LH (V)"=2.0, "U LH Lag (sec)"=0.06, "US (V)"=0.5, "US Lag (sec)"=0.15, "LH Position"=5.0, "Motor Resistance (Ohms)"=2.4, "Position Fault Thresh"=10.0} ("Control Cal In"), "TLead (sec)"=w114, "TLag (sec)"=w115, "KRpos (V/ )"=w116, "TIpos (sec)"=w117, "TDpos (sec)"=w118, "KRneg (V/ )"=w119, "TIneg (sec)"=w120, "TDneg (sec)"=w121, "LH Position Band"=w122, "U LH (V)"=w123, "U LH Lag (sec)"=w124, "US (V)"=w52, "US Lag (sec)"=w51, "LH Position"=w50, "Motor Resistance (Ohms)"=w49, "Position Fault Thresh"=w29) -> (w28:T28)
      n50 = Bundle By Name(cluster=T30 {"Analog1 Range (V)"=[0.0, 5.0], "Analog2 Range (V)"=[5.0, 0.0], "Position Range"=[0.0, 100.0]} ("Position Cal In"), "Analog1 Range (V)"=w95, "Analog2 Range (V)"=w94, "Position Range"=w93) -> (w110:T30)
      n51 = xnode "Read/Write Control"("FPGA VI Reference In"=w27) -> ("FPGA VI Reference Out"=w48:refnum<k20>, "Throttle-1.Data"=w38:T33)  [unwired: 1 in, 1 out]
      n52 = call <vilib>:"throttle_rt_data_convert_revb2.vi"("dt (sec)"=w23, "ThrottleDataFromFPGA"=w38) -> ("ThrottleDataToControl"=w18:T34)
      n53 = Unbundle By Name(w18) -> ("H1Sense (A)"=w47:sgl, "H2Sense (A)"=w46:sgl, "Analog1 (V)"=w45:sgl, "Analog2 (V)"=w44:sgl, "Battery (V)"=w43:sgl, "Temperature (C)"=w42:sgl, "ModulePresent"=w39:bool, "H1Fault"=w41:bool, "H2Fault"=w40:bool)
      n54 = call "Hardware|Throttle-1|ModeRequest"() -> ("Value"=w34:u32)
      n55 = call "Route Throttle AIs.vi"("ThrottleDataToControl"=w18, "ExternalAI1"="ExternalAI1 (optional)", "ExternalAI2"="ExternalAI2 (optional)", "UseExtAI1"=w17, "UseExtAI2"=w16) -> ("ThrottleDataToControl"=w19:T34)  [unwired: 10 in]
      n56 = To Unsigned Word Integer(number=w34) -> (unsigned 16bit integer=w24:u16)
      n57 = call "Hardware|Throttle-1|Ch1Freq"() -> ("Value"=w86:sgl)
      n58 = call "Hardware|Throttle-1|Init"() -> ("Value"=w126:bool)
      n59 = Type Cast(type=Mode_Request."IDLE" ("Mode Request"), x=w24) -> (*(type *) &x=w35:T29)
      n60 = call "Hardware|Throttle-1|PrimaryPsnSwitch"() -> ("Value"=w81:bool)
      n61 = call "Hardware|Throttle-1|Ch2Enable"() -> ("Value"=w88:bool)
      n62 = call "Hardware|Throttle-1|Ch2Freq"() -> ("Value"=w87:sgl)
      n63 = call "Hardware|Throttle-1|H1Sense"("Value"=w47) -> ()
      n64 = call "Hardware|Throttle-1|H2Sense"("Value"=w46) -> ()
      n65 = call "Hardware|Throttle-1|Analog1"("Value"=w45) -> ()
      n66 = call "Hardware|Throttle-1|Analog2"("Value"=w44) -> ()
      n67 = call "Hardware|Throttle-1|Battery"("Value"=w43) -> ()
      n68 = call "Hardware|Throttle-1|Temperature"("Value"=w42) -> ()
      n69 = call "Hardware|Throttle-1|ModulePresent"("Value"=w39) -> ()
      n70 = call "Hardware|Throttle-1|H1Fault"("Value"=w41) -> ()
      n71 = call "Hardware|Throttle-1|H2Fault"("Value"=w40) -> ()
      n72 = call "Critical|Throttle-1|H1Fault"("Fault"=w41) -> ()  [unwired: 2 in]
      n73 = call "Critical|Throttle-1|H2Fault"("Fault"=w40) -> ()  [unwired: 2 in]
      n74 = call <vilib>:"throttle_rt_control_revb2.vi"("Mode Request"=w35, "Module Data"=w19, "Primary Position (F=1, T=2)"=w81, "PWM Frequency (Hz)"=w86, "Position Setpoint"=w22, "dt (sec)"=w23, "Position Cal Settings"=w112, "Control Cal Settings"=cluster{"Control Calibration Setting":sgl} {"Control Calibration Setting"=0.0}, "Position Cal In"=w110, "Control Cal In"=w28, "initialize"=w126) -> ("Position Cal Out"=w109:T35, "Control Cal Out"=w108:T28, "Mode Status"=w32:T36, "Control Data"=w107:T37, "Throttle Period Ticks"=w92:u16, "Throttle Pulse Width Ticks"=w91:i16)  [unwired: 3 in]
      n75 = call "Hardware|Throttle-1|Ch2DutyCyc_Des"("Value"=w21) -> ()
      n76 = case shown="True" w88 {
        tunnel: [w135 w136] -> w90
        tunnel: [w135 w137] -> w89
        tunnel: w21 -> [_ w137]
        tunnel: w87 -> [_ w136]
        frame False {
          w135 = sgl 0.0 ("Value")
        }
        frame True {
        }
      }
      n77 = call <vilib>:"throttle2ticks_revb.vi"("DutyCycle (%)"=w89, "Frequency (Hz)"=w90) -> ("ThrottlePulseWidthTicks"=w134:i16, "ThrottlePeriodTicks"=w133:u16)
      n78 = To Unsigned Long Integer(number=w32) -> (unsigned 32bit integer=w31:u32)
      n79 = Unbundle By Name(w109) -> ("Primary Analog Range (V)"=w76:sgl[], "Secondary Analog Range (V)"=w77:sgl[], "Position Range"=w75:sgl[], "Position Calibrated"=w74:bool, "u Pos Cal Positive (V)"=w73:sgl, "u Pos Cal Negative (V)"=w72:sgl, "u Limit Positive"=w71:bool, "u Limit Negative"=w70:bool, "Pos Cal Diff Fault"=w69:bool)
      n80 = Unbundle By Name(w108) -> ("TLead (sec)"=w59:sgl, "TLag (sec)"=w58:sgl, "KRpos (V/ )"=w57:sgl, "TIpos (sec)"=w56:sgl, "TDpos (sec)"=w55:sgl, "KRneg (V/ )"=w54:sgl, "TIneg (sec)"=w53:sgl, "TDneg (sec)"=w68:sgl, "LH Position Band"=w67:sgl, "U LH (V)"=w66:sgl, "U LH Lag (sec)"=w65:sgl, "US (V)"=w64:sgl, "US Lag (sec)"=w63:sgl, "LH Position"=w62:sgl, "Motor Resistance (Ohms)"=w61:sgl, "Position Fault Thresh"=w60:sgl)
      n81 = Unbundle By Name(w107) -> ("Primary Position"=w37:sgl, "Secondary Position"=w36:sgl, "AboveLH?"=w80:bool, "Position Fault"=w79:bool, "u Limit?"=w78:bool, "uLHc (V)"=w85:sgl, "uFc (V)"=w84:sgl, "uPID (V)"=w83:sgl, "u (V)"=w82:sgl)
      n82 = call "Hardware|Throttle-1|ModeStatus"("Value"=w31) -> ()
      n83 = call "Hardware|Throttle-1|PrimaryPsn"("Value"=w37) -> ()
      n84 = call "Hardware|Throttle-1|SecondaryPsn"("Value"=w36) -> ()
      n85 = call "Hardware|Throttle-1|AboveLH"("Value"=w80) -> ()
      n86 = call "Hardware|Throttle-1|Psn_Fault"("Value"=w79) -> ()
      n87 = call "Hardware|Throttle-1|uLimit"("Value"=w78) -> ()
      n88 = call "Hardware|Throttle-1|uLHc"("Value"=w85) -> ()
      n89 = call "Hardware|Throttle-1|uFc"("Value"=w84) -> ()
      n90 = call "Hardware|Throttle-1|uPID"("Value"=w83) -> ()
      n91 = call "Hardware|Throttle-1|u"("Value"=w82) -> ()
      n92 = call "Hardware|Throttle-1|Ch1Enable"() -> ("Value"=w127:bool)
      n93 = call "Hardware|Throttle-1|TLead_Out"("Value"=w59) -> ()
      n94 = call "Hardware|Throttle-1|TLag_Out"("Value"=w58) -> ()
      n95 = call "Hardware|Throttle-1|KRPos_Out"("Value"=w57) -> ()
      n96 = call "Hardware|Throttle-1|TIPos_Out"("Value"=w56) -> ()
      n97 = call "Hardware|Throttle-1|TDPos_Out"("Value"=w55) -> ()
      n98 = call "Hardware|Throttle-1|KRNeg_Out"("Value"=w54) -> ()
      n99 = call "Hardware|Throttle-1|TINeg_Out"("Value"=w53) -> ()
      n100 = call "Hardware|Throttle-1|TDNeg_Out"("Value"=w68) -> ()
      n101 = call "Hardware|Throttle-1|LHPsnBand_Out"("Value"=w67) -> ()
      n102 = call "Hardware|Throttle-1|ULH_Out"("Value"=w66) -> ()
      n103 = call "Hardware|Throttle-1|ULHLag_Out"("Value"=w65) -> ()
      n104 = call "Hardware|Throttle-1|US_Out"("Value"=w64) -> ()
      n105 = call "Hardware|Throttle-1|USLag_Out"("Value"=w63) -> ()
      n106 = call "Hardware|Throttle-1|LHPsn_Out"("Value"=w62) -> ()
      n107 = call "Hardware|Throttle-1|MotorResistance_Out"("Value"=w61) -> ()
      n108 = call "Hardware|Throttle-1|Psn_FaultThreshOut"("Value"=w60) -> ()
      n109 = call "Hardware|Throttle-1|PrimaryAnalogRange"("Value"=w76) -> ()
      n110 = call "Hardware|Throttle-1|SecondaryAnalogRange"("Value"=w77) -> ()
      n111 = call "Hardware|Throttle-1|PsnRange_Out"("Value"=w75) -> ()
      n112 = call "Hardware|Throttle-1|PsnCalComplete"("Value"=w74) -> ()
      n113 = call "Hardware|Throttle-1|uPsnCalPos"("Value"=w73) -> ()
      n114 = call "Hardware|Throttle-1|uPsnCalNeg"("Value"=w72) -> ()
      n115 = call "Hardware|Throttle-1|uLimitPos"("Value"=w71) -> ()
      n116 = call "Hardware|Throttle-1|uLimitNeg"("Value"=w70) -> ()
      n117 = call "Hardware|Throttle-1|PsnCalDiff_Fault"("Value"=w69) -> ()
      n118 = case shown="True" w127 {
        tunnel: w92 -> [_ w139]
        tunnel: [w138 w140] -> w25
        tunnel: w91 -> [_ w140]
        tunnel: [w138 w139] -> w26
        frame False {
          w138 = i16 0 ("Throttle Pulse Width Ticks")
        }
        frame True {
        }
      }
      n119 = call "Hardware|Throttle-1|ModuleEnable"() -> ("Value"=w128:bool)
      n120 = feedback #3() -> (w129:bool)  [unwired: 1 in]
      n121 = Not(x=w129) -> (.not. x?=w130:bool)
      n122 = feedback-in #3(w130) -> ()
      n123 = Bundle By Name(cluster=T32 {"ModuleEnable"=FALSE, "WatchdogIn"=FALSE, "ThrottlePeriod"=0, "Throttle2Period"=0, "ThrottlePulseWidth"=0, "Throttle2PulseWidth"=0} ("ThrottleControl"), "ModuleEnable"=w128, "WatchdogIn"=w130, "ThrottlePulseWidth"=w25, "ThrottlePeriod"=w26, "Throttle2Period"=w133, "Throttle2PulseWidth"=w134) -> (w132:T32)
      n124 = xnode "Read/Write Control"("FPGA VI Reference In"=w48, "Throttle-1.Control"=w132) -> ()  [unwired: 1 in, 2 out]
    }
    frame Error {
    }
  }
  n125 = call "Hardware|Throttle-1|FPGAInterfaceError"("Value"=w1) -> ()
  n126 = call "Non-critical|Throttle-1|FPGAInterfaceError"("Fault"=w1) -> ()  [unwired: 2 in]
